vi "AllowRTEToRunSourceOnlyVIs.vi"() -> (0 "error out":errorcluster)   [LabVIEW 2012]
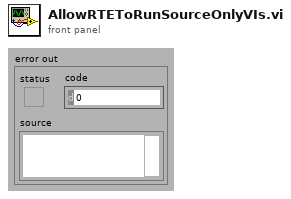
[diagram p1: front panel]
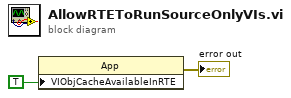
[diagram p0: block diagram]
diagram:
  n1 = property class="App"("VIObjCacheAvailableInRTE"=TRUE ("VIObjCache:Available in RTE")) -> (error out=→"error out":errorcluster)  [unwired: 2 in, 1 out]
